vi "file formatter.vi"() -> ()   [LabVIEW 2013]
uses:
  <vilib>/Utility/file.llb/Read From Spreadsheet File (string).vi
  <vilib>/Utility/file.llb/Write To Spreadsheet File (string).vi
panel:
  out "data string":string
  in  "Data Fields":T1={"Sphere"="", "Spectrometer"="", "Power Supply"="", "Analyzer"="", "Flicker"="", "Sample number"="", "Run time hours"=".csv", "Lamp Type"="", "Test orientation"="", "Source type"="", "Fixture type"="", "Project"="", "Measurement Type"="", "Operator Name"=""}
  # "ambient temp (sphere)"
  # "ambient temp room"
  # "Fill out the follow data fields for each test. An error will be thrown if any data fields are missing.\nNew parameters for data fields can be added by right clicking, hitting \"properties\", then \"edit items\""
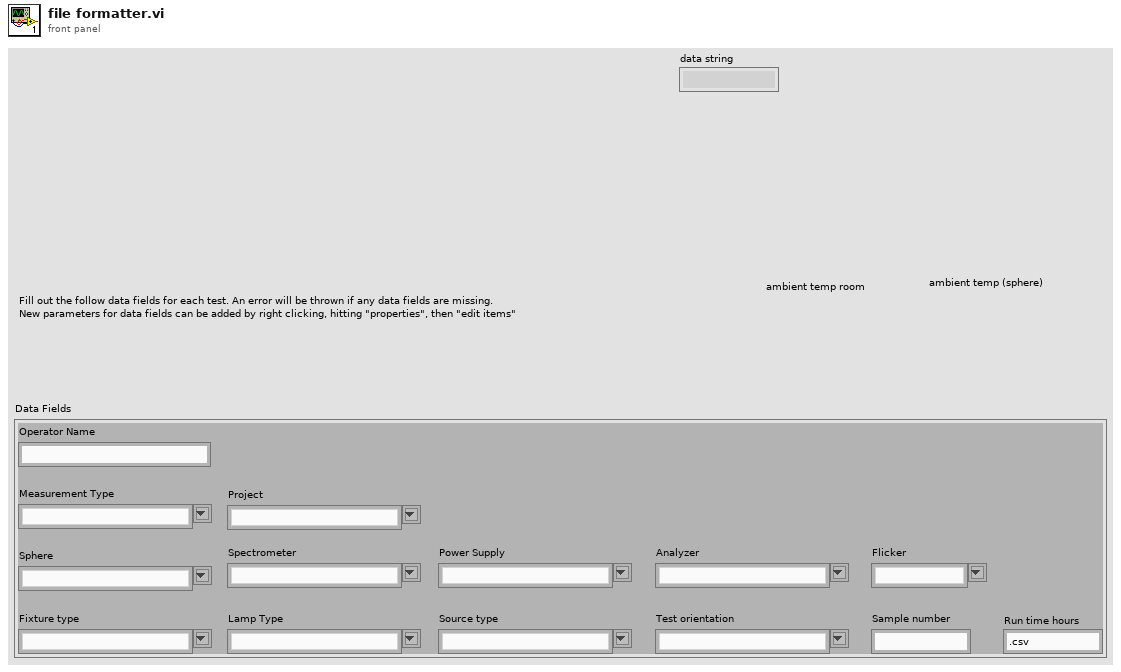
[diagram p1: front panel]
types:
  T1 = cluster{"Sphere":string, "Spectrometer":string, "Power Supply":string, "Analyzer":string, "Flicker":string, "Sample number":string, "Run time hours":string, "Lamp Type":string, "Test orientation":string, "Source type":string, "Fixture type":string, "Project":string, "Measurement Type":string, "Operator Name":string}
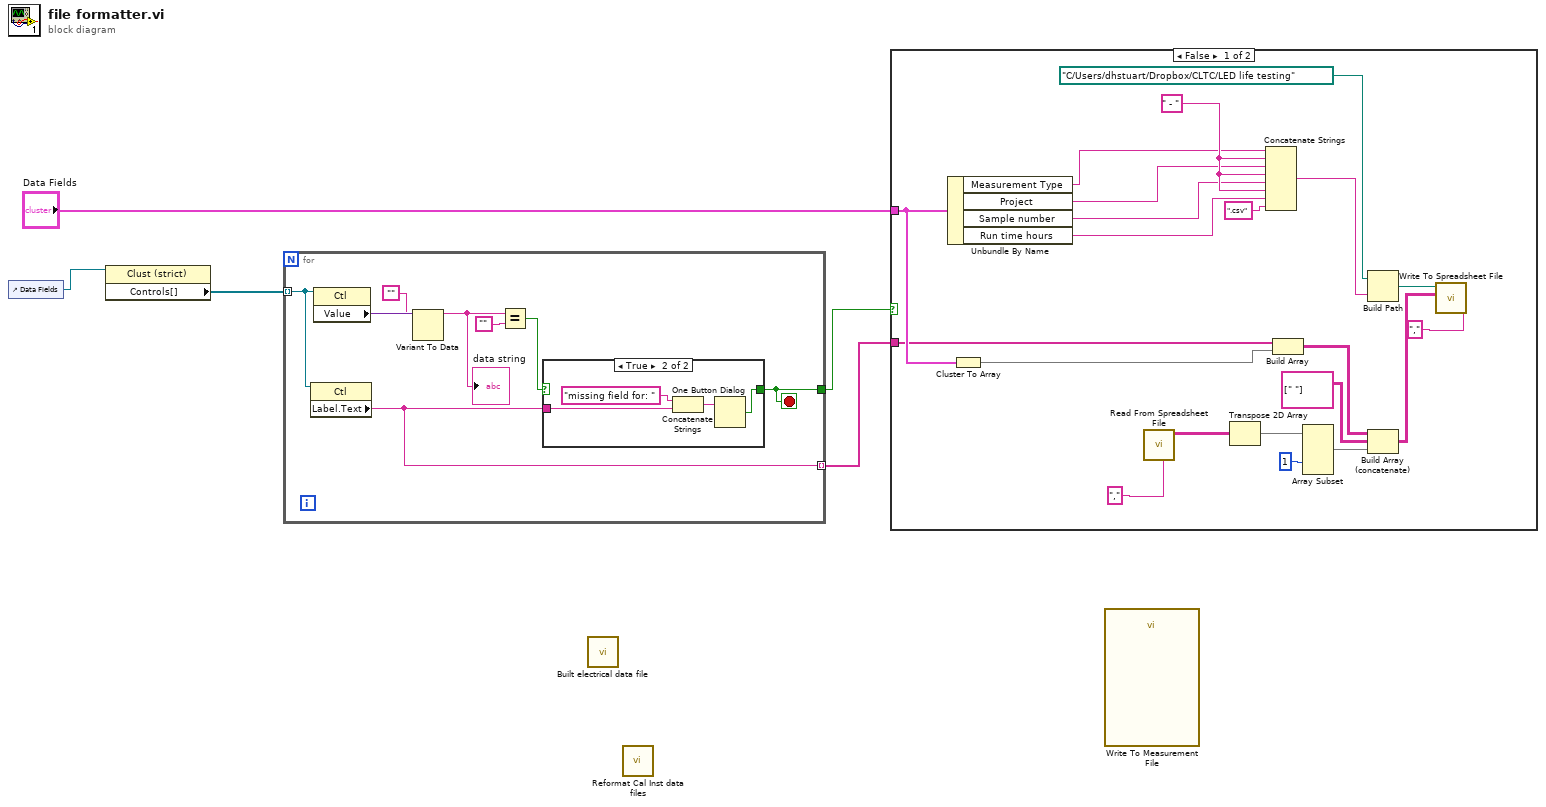
[diagram p0: block diagram]
diagram:
  n1 = control-ref of="Data Fields"() -> (w5:refnum<vi>)
  n2 = property class="Clust (strict)"(reference=w5) -> ("Controls[]"=w4:refnum<vi>[])  [unwired: 1 in, 2 out]
  n3 = for {
    tunnel: w4 -> [w9] mode=indexing
    tunnel: [w13] -> w3
    tunnel: [w6] -> w1 mode=indexing
    stop <- w13 stop-if-true
    n4 = property class="Ctl"(reference=w9) -> ("Label.Text"=w6:string)  [unwired: 1 in, 2 out]
    n5 = property class="Ctl"(reference=w9) -> ("Value"=w11:variant)  [unwired: 1 in, 2 out]
    n6 = Variant To Data(type="", Variant=w11) -> (data=w10:string)  [unwired: 1 in, 1 out]
    "data string" <- w10
    n7 = Equal?(x=w10, y="") -> (x = y?=w12:bool)
    n8 = case shown="True" w12 {
      selector: w12 -> [w14 _]
      tunnel: w6 -> [_ w17]
      tunnel: [w14 w15] -> w13
      frame False {
      }
      frame True {
        n9 = Concatenate Strings("missing field for: ", w17) -> (w16:string)
        n10 = One Button Dialog(message=w16) -> (true=w15:bool)  [unwired: 1 in]
      }
    }
  }
  n11 = call "Built electrical data file.vi"() -> ()  [unwired: 11 in, 1 out]
  n12 = call "Reformat Cal Inst data files.vi"() -> ()  [unwired: 11 in, 1 out]
  n13 = case shown="False" w3 {
    tunnel: "Data Fields" -> [w25 _]
    tunnel: w1 -> [w24 _]
    frame False {
      w39 = " - "
      n14 = Unbundle By Name(w25) -> ("Measurement Type"=w22:string, "Project"=w21:string, "Sample number"=w20:string, "Run time hours"=w19:string)
      n15 = Cluster To Array(cluster=w25) -> (array=w23:string[])
      n16 = call-poly <vilib>:"Read From Spreadsheet File.vi"("delimiter (\\t)"="," ("delimiter (\\t)")) -> ("all rows"=w36:string[][])  [unwired: 6 in, 4 out]
      n17 = Transpose 2D Array(2D array=w36) -> (transposed array=w31:string[][])
      n18 = Concatenate Strings(w22, w39, w21, w39, w20, w39, w19, ".csv" ("string")) -> (w27:string)
      n19 = Build Array(w24, w23) -> (w37:string[][])
      n20 = Array Subset(array=w31, index (col)=1 ("index")) -> (w30:string[][])  [unwired: 3 in]
      n21 = Build Path(base path=path "C:/Users/dhstuart/Dropbox/CLTC/LED life testing" ("file path (dialog if empty)"), name or relative path=w27) -> (appended path=w26:path)
      n22 = Build Array (concatenate)(w37, string[][] [[" "]] ("array"), w30) -> (w34:string[][])
      n23 = call-poly <vilib>:"Write To Spreadsheet File.vi"("delimiter (\\t)"="," ("delimiter (\\t)"), "2D data"=w34, "file path (dialog if empty)"=w26) -> ()  [unwired: 5 in, 1 out]
    }
    frame True {
    }
  }
  n24 = call "Write To Measurement File"() -> ()  [unwired: 17 in, 3 out]
